vi "Enqueue SelfQueue Msg.vi"(8 "error in (no error)":errorcluster, 9 "Message Data":variant, 10 "Message":string, 11 "ModuleAbstract in":refnum<class "ModuleAbstract.lvclass">) -> (0 "error out":errorcluster, 3 "ModuleAbstract out":refnum<class "ModuleAbstract.lvclass">)   [LabVIEW 2019, in "ModuleAbstract.lvlib" / "ModuleAbstract.lvclass"]
uses:
  ModuleAbstract.lvclass
  ModuleAbstract.lvclass/ModuleAbstract.ctl
  Utilities/LV_Lib/Message Queue/Enqueue Message (Single).vi
  Utilities/LV_Lib/Message Queue/Message Queue.lvlib
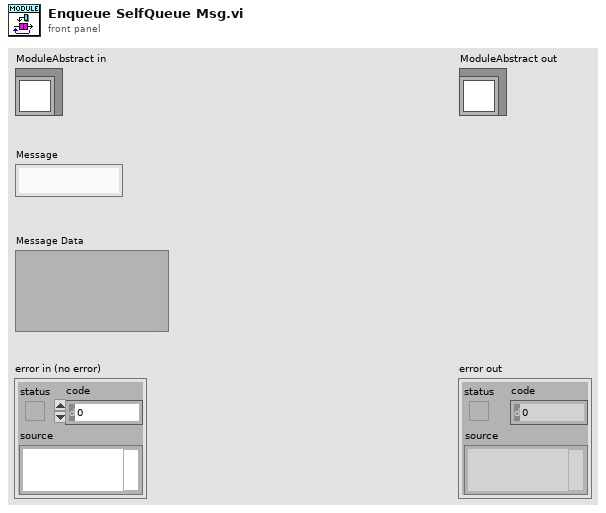
[diagram p1: front panel]
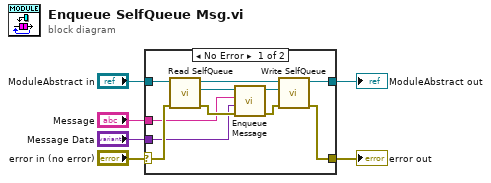
[diagram p0: block diagram]
diagram:
  n1 = case shown="No Error" "error in (no error)" {
    selector: "error in (no error)" -> [w10 w19]
    tunnel: [w9 w19] -> w5
    tunnel: [w11 w18] -> w3
    tunnel: "ModuleAbstract in" -> [w12 w18]
    tunnel: "Message" -> [w8 _]
    tunnel: "Message Data" -> [w7 _]
    frame No Error {
      n2 = call "Read SelfQueue.vi"("error in (no error)"=w10, "ModuleAbstract in"=w12) -> ("error out"=w14:errorcluster, "SelfQueue"=w17:refnum<queue>, "ModuleAbstract out"=w15:refnum<class "ModuleAbstract.lvclass">)  [unwired: 7 in]
      n3 = call-poly "Enqueue Message.vi"("error in (no error)"=w14, "Message Data"=w7, "Message"=w8, "Message Queue"=w17) -> ("error out"=w13:errorcluster, "dup Message Queue"=w16:refnum<queue>)  [unwired: 6 in]
      n4 = call "Write SelfQueue.vi"("error in (no error)"=w13, "SelfQueue"=w16, "ModuleAbstract in"=w15) -> ("error out"=w9:errorcluster, "ModuleAbstract out"=w11:refnum<class "ModuleAbstract.lvclass">)  [unwired: 7 in]
    }
    frame Error {
    }
  }
  "error out" <- w5
  "ModuleAbstract out" <- w3
